vi "niSwitch DMM Switch Synchronous Scanning.vi"() -> ()   [LabVIEW 2011]
doc: "I. Description:\n\nThis example demonstrates how to scan a series of channels on a switch module and take measurements with an NI digital multimeter using synchronous scanning. \n\nSYNCHRONOUS SCANNING:\nThe DMM takes a measurement and generates a digital pulse-Measurement Complete (MC). When the switch receives this digital pulse, it advances to the next entry in its scan list. The DMM takes the next measurement after a time interval. You must program the DMM interval time by configuring an Interval Sample Trigger. Set the Interval parameter to, at least, the time needed for the switch to activate and settle. \n\nII. Instructions for Running:\n\nTo make this example work with your switch, complete the following:\nSWITCH SETUP: (refer to the NI Switches Help) \n1) Enter the DAQmx/traditional DAQ switch resource name.\n2) Select the correct topology for your switch module.\n3) Enter a valid scan list.\n3) Select a valid value for Trigger Input. \n\nDMM SETUP: (refer to your NI DMM documentation)\n1) Enter your traditional DAQ DMM resource name.\n2) Select measurement type, range and resolution.\n3) Enter number of samples and sample interval.\n4) Select a valid MC destination.\n\nRefer to the NI Switches Help to determine if your switch supports scanning, the scan list syntax, and the valid channel names and valid resource names for your switch module.\n\nIII. Block Diagram Steps:\n\nA) The switch is configured first. Triggers and scan list are set. \nB) The DMM is configured. Functions, range, resolution, triggers and number of points to take are set. \nC) When the switch initiates, it connects the first channel in its scan list, enters the wait for trigger state, and allows the rest of the program to continue. \nD) When the DMM initiates it configures its hardware according to the settings from step B) and takes a measurement. This measures the first connection in the switch scan list. The DMM sends its MC signal to the switch to advance to the next connection. Then the switch moves to the next entry in its scan list and waits for a new trigger. The DMM then takes a new measurement after the interval time set in Sample interval parameter has elapsed. This operation repeats until the number of measurements is equal to the Sample Count. When all the points have been acquired, they are returned to the user (fetch) and the DMM session is closed.\nE) Terminates the scanning operation, closes the session to the switch, and displays errors if any.\n\nIV. I/O Connections Overview:\n\nRefer to the NI Switches Getting Started Guide and NI Switches Help for information about connecting signals to your switch module."
uses:
  <instrlib>/niSwitch/niSwitch.LLB/niSwitch Topologies.ctl
  <instrlib>/niDMM/nidmm.llb/niDMM Function.ctl
  <instrlib>/niSwitch/niSwitch.LLB/niSwitch Scan Advanced Output.ctl
  <instrlib>/niDMM/nidmm.llb/niDMM Sample Trigger.ctl
panel:
  in  "measurement complete destination":u16(ring)=2 items=["None", "External", "TTL 0", "TTL 1", "TTL 2", "TTL 3", "TTL 4", "TTL 5", "TTL 6", "TTL 7", "LBR Trig 0"]
  in  "measurement type":T1
  in  "topology name":T2="2503/2-Wire 24x1 Mux"
  in  "resource name":refnum<k15>="SWITCH"
  in  "scan list":string="ch0:5->com0;"
  in  "trigger input":T3(ring)=enum."TTL0"
  in  "resolution":dbl=0.0001 format="%.0p"
  in  "resource name":refnum<k15>="DMM"
  in  "sample count":i32=10
  in  "sample interval (sec)":dbl=0.1 format="%.2f"
  in  "range":dbl=10.0 format="%.2f"
  out "Measurements":dbl[](graph)
  # "SWITCH"
  # "DMM"
  # "For instructions, select File >> VI Properties >> Documentation."
  # "For a list of valid switch channel names, select Help >> NI Switches Help >> Devices Overview >> [Module Number]"
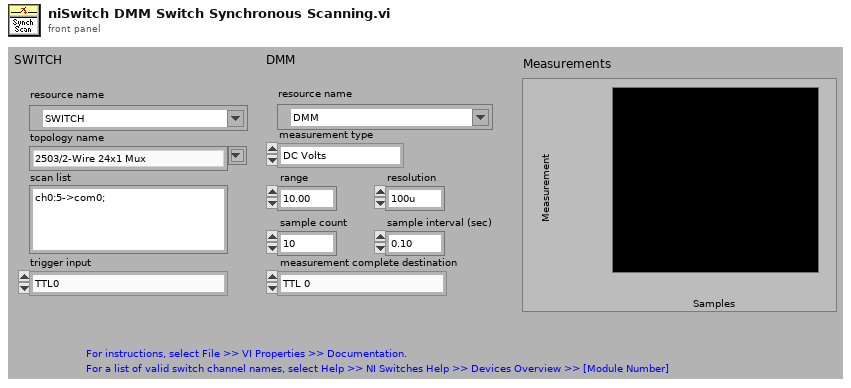
[diagram p1: front panel]
types:
  T1 = typedef "niDMM Function.ctl" = enum16{"DC Volts", "AC Volts", "DC Current", "AC Current", "2-wire Resistance", "4-wire Resistance", "Diode", "Frequency", "Period", "AC Volts DC Coupled", "Capacitance", "Inductance", "Temperature"}
  T2 = typedef "niSwitch Topologies.ctl" = string
  T3 = enum16{"Immediate", "External", "TTL0", "TTL1", "TTL2", "TTL3", "TTL4", "TTL5", "TTL6", "TTL7", "ECL0", "ECL1", "PXI Star", "Software Trigger Function", "Rear Connector", "Front Connector", "Rear Connector of Module 1", "Rear Connector of Module 2", "Rear Connector of Module 3", "Rear Connector of Module 4", "Rear Connector of Module 5", "Rear Connector of Module 6", "Rear Connector of Module 7", "Rear Connector of Module 8", "Rear Connector of Module 9", "Rear Connector of Module 10", "Rear Connector of Module 11", "Rear Connector of Module 12", "Front Connector of Module 1", "Front Connector of Module 2", "Front Connector of Module 3", "Front Connector of Module 4", "Front Connector of Module 5", "Front Connector of Module 6", "Front Connector of Module 7", "Front Connector of Module 8", "Front Connector of Module 9", "Front Connector of Module 10", "Front Connector of Module 11", "Front Connector of Module 12"}
  T4 = typedef "niDMM Sample Trigger.ctl" = enum16{"Immediate", "External", "TTL 0", "TTL 1", "TTL 2", "TTL 3", "TTL 4", "TTL 5", "TTL 6", "Interval", "Software", "TTL 7", "PXI Star", "LBR Trig 1", "Aux Trig 1"}
  T5 = typedef "niSwitch Scan Advanced Output.ctl" = enum16{"None", "External", "TTL0", "TTL1", "TTL2", "TTL3", "TTL4", "TTL5", "TTL6", "TTL7", "ECL0", "ECL1", "PXI Star", "Rear Connector", "Front Connector", "Rear Connector Module 1", "Rear Connector Module 2", "Rear Connector Module 3", "Rear Connector Module 4", "Rear Connector Module 5", "Rear Connector Module 6", "Rear Connector Module 7", "Rear Connector Module 8", "Rear Connector Module 9", "Rear Connector Module 10", "Rear Connector Module 11", "Rear Connector Module 12", "Front Connector Module 1", "Front Connector Module 2", "Front Connector Module 3", "Front Connector Module 4", "Front Connector Module 5", "Front Connector Module 6", "Front Connector Module 7", "Front Connector Module 8", "Front Connector Module 9", "Front Connector Module 10", "Front Connector Module 11", "Front Connector Module 12"}
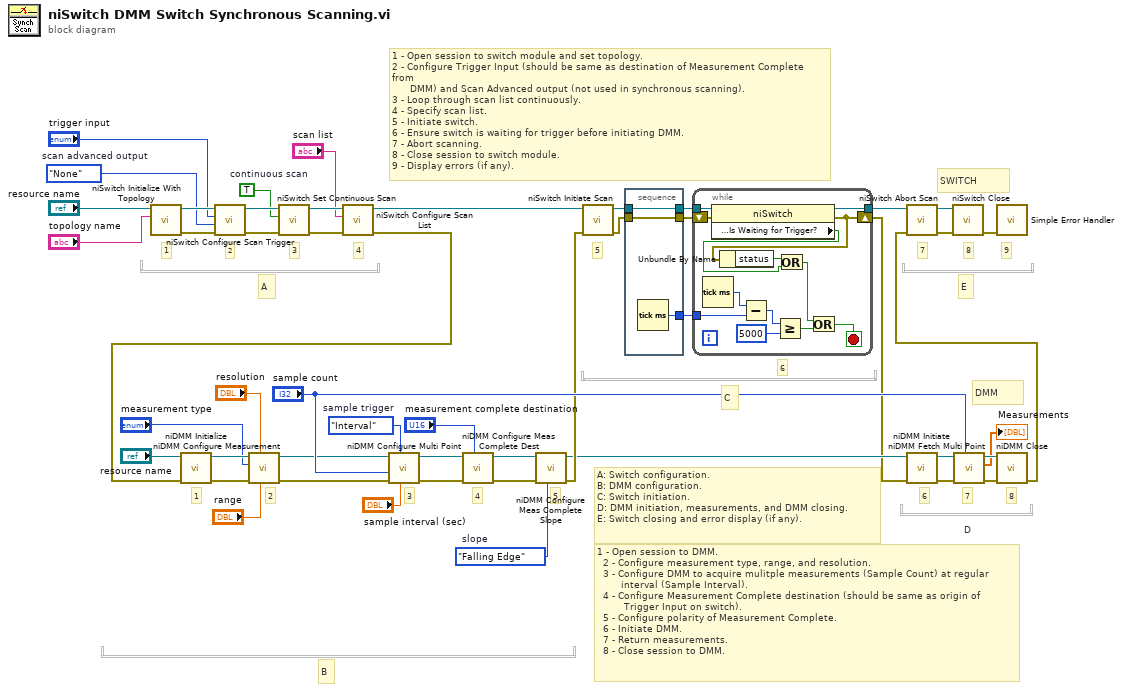
[diagram p0: block diagram]
diagram:
  w3 = niDMM_Sample_Trigger."Interval"  # sample trigger
  w16 = enum16{"Rising Edge", "Falling Edge"}."Falling Edge"  # slope
  w26 = niSwitch_Scan_Advanced_Output."None"  # scan advanced output
  w45 = TRUE  # continuous scan
  # "1 - Open session to switch module and set topology.\n2 - Configure Trigger Input (should be same as destination of Measurement Complete from\n      DMM) and Scan Advanced output (not used in synchronous scanning).\n3 - Loop through scan list continuously.\n4 - Specify scan list.\n5 - Initiate switch.\n6 - Ensure switch is waiting for trigger before initiating DMM. \n7 - Abort scanning.\n8 - Close session to switch module.\n9 - Display errors (if any)."
  # "A: Switch configuration.\nB: DMM configuration.\nC: Switch initiation.\nD: DMM initiation, measurements, and DMM closing.\nE: Switch closing and error display (if any)."
  # "8"
  # "E"
  # "D"
  # "C"
  # "B"
  # "A"
  # "7"
  # "5"
  # "DMM"
  # "SWITCH"
  # "4"
  # "1 - Open session to DMM.\n  2 - Configure measurement type, range, and resolution.\n  3 - Configure DMM to acquire mulitple measurements (Sample Count) at regular\n        interval (Sample Interval).\n  4 - Configure Measurement Complete destination (should be same as origin of\n         Trigger Input on switch).\n  5 - Configure polarity of Measurement Complete.\n  6 - Initiate DMM.\n  7 - Return measurements.\n  8 - Close session to DMM."
  # "1"
  # "6"
  # "3"
  # "2"
  # "6"
  # "9"
  # "8"
  # "7"
  # "5"
  # "4"
  # "3"
  # "2"
  # "1"
  n1 = call <instrlib>:"niSwitch Initialize With Topology.vi"("topology name"="topology name", "resource name"="resource name") -> ("error out"=w42:errorcluster, "instrument handle out"=w43:refnum<k15>)  [unwired: 8 in]
  n2 = call <instrlib>:"niSwitch Configure Scan Trigger.vi"("error in (no error)"=w42, "scan advanced output (External)"=w26, "trigger input (External)"="trigger input", "instrument handle"=w43) -> ("error out"=w46:errorcluster, "instrument handle out"=w48:refnum<k15>)  [unwired: 6 in]
  n3 = call <instrlib>:"niSwitch Set Continuous Scan.vi"("error in (no error)"=w46, "continuous scan (False)"=w45, "instrument handle"=w48) -> ("error out"=w40:errorcluster, "instrument handle out"=w41:refnum<k15>)  [unwired: 7 in]
  n4 = call <instrlib>:"niSwitch Configure Scan List.vi"("error in (no error)"=w40, "scan list"="scan list", "instrument handle"=w41) -> ("error out"=w21:errorcluster, "instrument handle out"=w22:refnum<k15>)  [unwired: 7 in]
  n5 = call <instrlib>:"niDMM Initialize.vi"("error in (no error)"=w21, "Instrument Descriptor"="resource name") -> ("error out"=w38:errorcluster, "instrument handle out"=w39:refnum<k15>)  [unwired: 8 in]
  n6 = call <instrlib>:"niDMM Configure Measurement.vi"("Range"="range", "Resolution"="resolution", "error in (no error)"=w38, "Function"="measurement type", "instrument handle"=w39) -> ("error out"=w15:errorcluster, "instrument handle out"=w14:refnum<k15>)  [unwired: 5 in]
  n7 = call <instrlib>:"niDMM Configure Multi Point.vi"("Sample Interval (sec)"="sample interval (sec)", "Sample Trigger"=w3, "error in (no error)"=w15, "Sample Count"="sample count", "instrument handle"=w14) -> ("error out"=w29:errorcluster, "instrument handle out"=w30:refnum<k15>)  [unwired: 5 in]
  n8 = call <instrlib>:"niDMM Configure Meas Complete Dest.vi"("Measurement Complete Destination"="measurement complete destination", "error in (no error)"=w29, "instrument handle"=w30) -> ("error out"=w20:errorcluster, "instrument handle out"=w19:refnum<k15>)  [unwired: 7 in]
  n9 = call <instrlib>:"niDMM Configure Meas Complete Slope.vi"("Slope"=w16, "error in (no error)"=w20, "instrument handle"=w19) -> ("error out"=w18:errorcluster, "instrument handle out"=w17:refnum<k15>)  [unwired: 7 in]
  n10 = call <instrlib>:"niSwitch Initiate Scan.vi"("error in (no error)"=w18, "instrument handle"=w22) -> ("error out"=w7:errorcluster, "instrument handle out"=w8:refnum<k15>)  [unwired: 8 in]
  n11 = stacked-sequence {
    tunnel: [w52] -> w13
    tunnel: w8 -> [w52]
    tunnel: [w51] -> w12
    tunnel: w7 -> [w51]
    tunnel: [w50] -> w11
    frame #0 {
      n12 = Tick Count (ms)() -> (millisecond timer value=w50:u32)
    }
  }
  n13 = while {
    tunnel: [w64] -> w9
    tunnel: w13 -> [w65]
    shift-right: [w60] -> w10
    shift-left: w12 -> [w59]
    tunnel: w11 -> [w54]
    stop <- w53 stop-if-true
    n14 = Tick Count (ms)() -> (millisecond timer value=w55:u32)
    n15 = property class="niSwitch"(reference=w65, error in=w59) -> (reference out=w64:refnum<k15>, error out=w60:errorcluster, "Scanning Configuration:Is Waiting for Trigger?"=w62:bool)
    n16 = Unbundle By Name(w60) -> ("status"=w63:bool)
    n17 = Subtract(x=w55, y=w54) -> (x-y=w57:u32)
    n18 = Greater Or Equal?(x=w57, y=u32 5000) -> (x >= y?=w56:bool)
    n19 = Or(x=w63, y=w62) -> (x .or. y?=w61:bool)
    n20 = Or(x=w61, y=w56) -> (x .or. y?=w53:bool)
  }
  n21 = call <instrlib>:"niDMM Initiate.vi"("error in (no error)"=w10, "instrument handle"=w17) -> ("error out"=w32:errorcluster, "instrument handle out"=w34:refnum<k15>)  [unwired: 8 in]
  n22 = call <instrlib>:"niDMM Fetch Multi Point.vi"("Number to Fetch"="sample count", "error in (no error)"=w32, "instrument handle"=w34) -> ("error out"=w31:errorcluster, "Measurements"=→"Measurements":dbl[], "instrument handle out"=w28:refnum<k15>)  [unwired: 5 in, 1 out]
  n23 = call <instrlib>:"niDMM Close.vi"("error in (no error)"=w31, "instrument handle"=w28) -> ("error out"=w6:errorcluster)  [unwired: 9 in]
  n24 = call <instrlib>:"niSwitch Abort Scan.vi"("error in (no error)"=w6, "instrument handle"=w9) -> ("error out"=w44:errorcluster, "instrument handle out"=w47:refnum<k15>)  [unwired: 8 in]
  n25 = call <instrlib>:"niSwitch Close.vi"("error in (no error)"=w44, "instrument handle"=w47) -> ("error out"=w49:errorcluster)  [unwired: 9 in]
  n26 = call <vilib>:"Simple Error Handler.vi"("error in (no error)"=w49) -> ()  [unwired: 4 in, 5 out]
